vi "Export Experiment Data.vi"(8 "uS Array":dbl[](array[numeric]), 9 "Skip Export":bool, 10 "Export?":bool, 11 "Data":dbl[][](array[numeric])) -> (3 "Export Complete?":bool)   [LabVIEW 2016]
uses:
  <vilib>/Utility/error.llb/DialogType.ctl
  <vilib>/Utility/file.llb/Write Delimited Spreadsheet (string).vi
  <vilib>/Utility/file.llb/Write Delimited Spreadsheet (DBL).vi
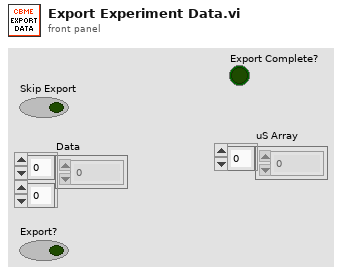
[diagram p1: front panel]
types:
  T1 = enum16{"open", "replace", "create", "open or create", "replace or create", "replace or create with confirmation"}
  T2 = typedef "DialogType.ctl" = u16
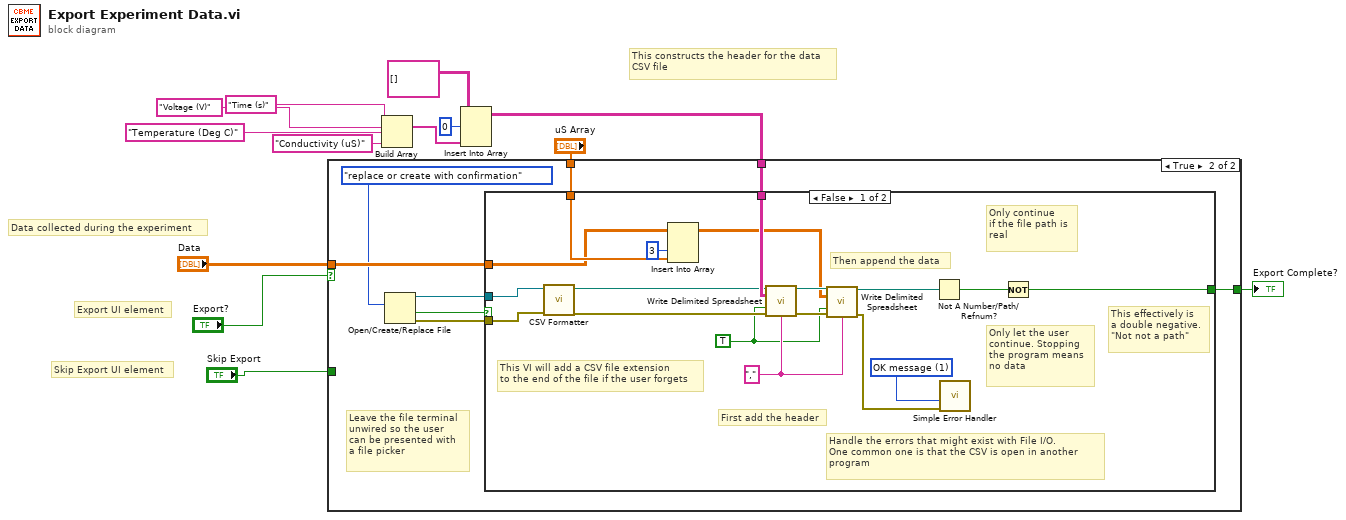
[diagram p0: block diagram]
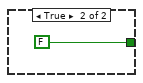
[diagram p3: hidden frame]
diagram:
  # "Skip Export UI element"
  # "Export UI element"
  # "Data collected during the experiment"
  # "This constructs the header for the data\nCSV file"
  n1 = Build Array("Time (s)", "Voltage (V)", "Temperature (Deg C)", "Conductivity (uS)" ("element")) -> (w8:string[])
  n2 = Insert Into Array(array=string[][] [], index (row)=0, new element=w8) -> (w11:string[][])  [unwired: 1 in]
  n3 = case shown="True" "Export?" {
    tunnel: "Data" -> [_ w21]
    tunnel: [w14 w22] -> w3
    tunnel: "Skip Export" -> [w14 _]
    tunnel: w11 -> [_ w20]
    tunnel: "uS Array" -> [_ w15]
    frame False {
      # "The user doesn't want to export,\nso skip this step"
    }
    frame True {
      # "Leave the file terminal \nunwired so the user \ncan be presented with \na file picker"
      n4 = Open/Create/Replace File(operation (0:open)=T1."replace or create with confirmation") -> (refnum out=w16:refnum<file>, cancelled=w18:bool, error out=w17:errorcluster)  [unwired: 5 in]
      n5 = case shown="False" w18 {
        tunnel: [w38 FALSE] -> w22
        tunnel: w21 -> [w24 _]
        tunnel: w20 -> [w35 _]
        tunnel: w17 -> [w31 _]
        tunnel: w16 -> [w30 _]
        tunnel: w15 -> [w26 _]
        frame False {
          w32 = T2 1 items=["no dialog", "OK message", "continue or stop message", "OK message + warnings", "continue/stop + warnings"] ("type of dialog (OK msg:1)")
          w28 = TRUE ("append to file? (new file:F)")
          w34 = "," ("delimiter (\\t)")
          # "This VI will add a CSV file extension\nto the end of the file if the user forgets"
          # "Only let the user\ncontinue. Stopping\nthe program means\nno data"
          # "Handle the errors that might exist with File I/O.\nOne common one is that the CSV is open in another\nprogram"
          # "This effectively is\na double negative.\n\"Not not a path\""
          # "Only continue\nif the file path is \nreal"
          # "Then append the data"
          # "First add the header"
          n6 = call "CSV Formatter.vi"("error in (no error)"=w31, "Byte Stream File in"=w30) -> ("error out"=w29:errorcluster, "path"=w27:path)  [unwired: 8 in]
          n7 = Insert Into Array(array=w24, index (col)=3 ("disabled index (col)"), new element=w26) -> (w23:dbl[][])  [unwired: 1 in]
          n8 = call-poly <vilib>:"Write Delimited Spreadsheet.vi"("file path (dialog if empty)"=w27, "2D data"=w35, "append to file? (new file:F)"=w28, "error in (no error)"=w29, "delimiter (\\t)"=w34) -> ("new file path (Not A Path if cancelled)"=w37:path, "error out"=w36:errorcluster)  [unwired: 9 in]
          n9 = call-poly <vilib>:"Write Delimited Spreadsheet.vi"("file path (dialog if empty)"=w37, "2D data"=w23, "append to file? (new file:F)"=w28, "error in (no error)"=w36, "delimiter (\\t)"=w34) -> ("new file path (Not A Path if cancelled)"=w40:path, "error out"=w33:errorcluster)  [unwired: 9 in]
          n10 = Not A Number/Path/Refnum?(number/path/refnum=w40) -> (NaN/Path/Refnum?=w39:bool)
          n11 = call <vilib>:"Simple Error Handler.vi"("type of dialog (OK msg:1)"=w32, "error in (no error)"=w33) -> ()  [unwired: 3 in, 5 out]
          n12 = Not(x=w39) -> (.not. x?=w38:bool)
        }
        frame True {
        }
      }
    }
  }
  "Export Complete?" <- w3
